vi "CountImpulse.vi"(8 "error in":errorcluster, 10 "stop (F)":bool, 11 "number of samples":i32=100) -> (0 "error out":errorcluster, 2 "stopped":bool, 3 "Ilość impulsów":dbl)   [LabVIEW 2021]
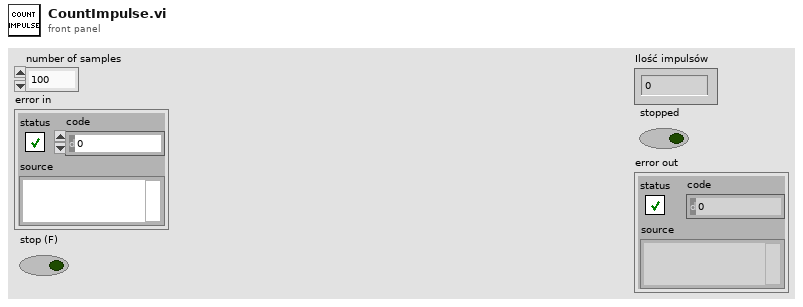
[diagram p1: front panel]
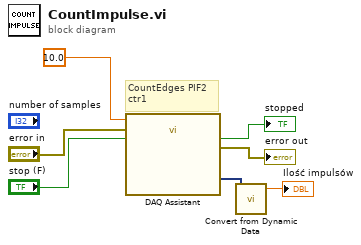
[diagram p0: block diagram]
diagram:
  # "CountEdges PIF2\nctr1"
  n1 = call "DAQ Assistant"("timeout (s)"=10.0, "error in"="error in", "stop (F)"="stop (F)") -> ("data"=w7:dynamicdata, "stopped"=→"stopped":bool, "error out"=→"error out":errorcluster)  [unwired: 13 in, 1 out]
  n2 = call "Convert from Dynamic Data"("Dynamic Data Type"=w7) -> ("Scalar"=→"Ilość impulsów":dbl)  [unwired: 3 in]
